vi "PCA_Probe.vi"(11 "OpenLvVision_OpenCv.lvlib:PCA":refnum<class "PCA.lvclass">) -> (2 "Value String":string, 3 "Pause VI":bool)   [LabVIEW 2020, in "OpenLvVision_OpenCv.lvlib" / "PCA.lvclass"]
uses:
  PCA.lvclass
  _LvHelpers/EdvrObject/EdvrObject.lvclass
  C:/Users/lukas/Downloads/OpenLvVision_OpenCv/SourceCode/LabView/OpenLvVision_OpenCv/_LvHelpers/EdvrObject/EdvrObject.lvclass
panel:
  in  "Tab Control":enum32{"EigenValues", "EigenVectors", "Mean"}(tab)
  out "EigenValues":dbl[](array[numeric])
  out "EigenVectors":dbl[][](array[numeric])
  out "Mean":dbl[][](array[numeric])
  out "Reference":u64 format="%.0x"
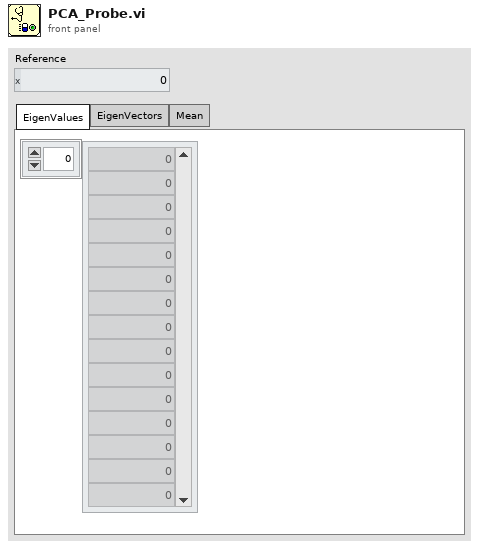
[diagram p1: front panel]
types:
  T1 = typedef "OpenLvVision_OpenCv.lvlib/EdvrObject.lvclass/Edvr.ctl" = refnum<data-value>
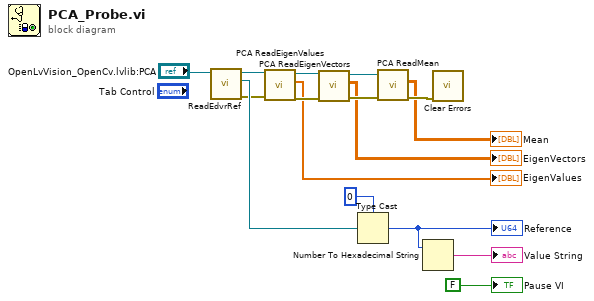
[diagram p0: block diagram]
diagram:
  n1 = call "ReadEdvrRef.vi"("EdvrObject in"="OpenLvVision_OpenCv.lvlib:PCA") -> ("error out"=w11:errorcluster, "Edvr"=w14:T1, "EdvrObject out"=w12:refnum<class "PCA.lvclass">)  [unwired: 8 in]
  n2 = call "PCA ReadEigenValues.vi"("error in (no error)"=w11, "PCA in"=w12) -> ("error out"=w9:errorcluster, "EigenValues"=→"EigenValues":dbl[], "PCA out"=w10:refnum<class "PCA.lvclass">)  [unwired: 7 in]
  n3 = call "PCA ReadEigenVectors.vi"("error in (no error)"=w9, "PCA in"=w10) -> ("error out"=w7:errorcluster, "EigenVectors"=→"EigenVectors":dbl[][], "PCA out"=w8:refnum<class "PCA.lvclass">)  [unwired: 7 in]
  n4 = Type Cast(type=u64 0, x=w14) -> (*(type *) &x=w2:u64)
  "Reference" <- w2
  n5 = call "PCA ReadMean.vi"("error in (no error)"=w7, "PCA in"=w8) -> ("error out"=w6:errorcluster, "Mean"=→"Mean":dbl[][])  [unwired: 7 in, 1 out]
  n6 = Number To Hexadecimal String(2:w2) -> (0:→"Value String":string)  [unwired: 1 in]
  n7 = call <vilib>:"Clear Errors.vi"("error in (no error)"=w6) -> ()  [unwired: 5 in, 2 out]
  "Pause VI" <- FALSE
